vi "Pre Launch Init.vi"(11 "Base UI Actor in":refnum<class "Base UI Actor.lvclass">) -> (0 "error out":errorcluster, 3 "Base UI Actor out":refnum<class "Base UI Actor.lvclass">)   [LabVIEW 2020, in "Base UI Actor.lvlib" / "Base UI Actor.lvclass"]
doc: "(<B>Filename</B>: Actor Framework.lvlib:Actor.lvclass:Pre Launch Init.vi)\n\nDefines behavior that occurs after the Launch Nested Actor method is invoked but before the actor's Actor Core method begins running.\n\nBy default, this method does nothing. A descendant class may override it to define behavior."
uses:
  Base UI Actor.lvclass
  <vilib>/ActorFramework/Actor/Actor.lvclass
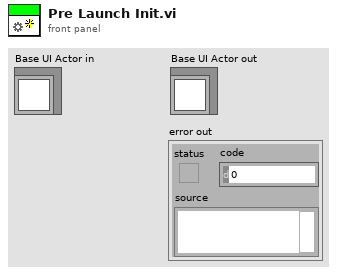
[diagram p1: front panel]
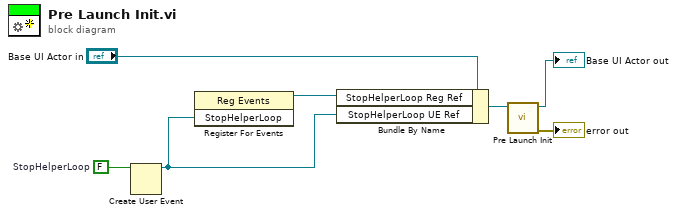
[diagram p0: block diagram]
diagram:
  w4 = FALSE  # StopHelperLoop
  n1 = Create User Event(user event datatype=w4) -> (user event=w1:refnum<user-event>)  [unwired: 1 in, 1 out]
  n2 = register-events(w1) -> (reference out=w2:refnum<event-registration>)  [unwired: 2 in, 1 out]
  n3 = Bundle By Name(cluster="Base UI Actor in", "StopHelperLoop Reg Ref"=w2, "StopHelperLoop UE Ref"=w1) -> (w3:refnum<class "Base UI Actor.lvclass">)
  n4 = call-parent "Pre Launch Init.vi"("Actor in"=w3) -> ("error out"=→"error out":errorcluster, "Actor out"=→"Base UI Actor out":refnum<class "Base UI Actor.lvclass">)  [unwired: 9 in]
